vi "Begin.vi"(8 "error in":errorcluster) -> (0 "error out":errorcluster)   [LabVIEW 2018]
doc: "Called before other user functions, this VI is expected to open initial I/O refnums, load in file data, and do all program initialization. Notice that the <B>error out</B> terminal is simply used for data flow. Wiring it to other structures or subVIs ensures that this VI runs first."
uses:
  <vilib>/Rock Robotics/WPI/DriverStation/WPI_DriverStationRobotMode2.ctl
  <vilib>/Rock Robotics/WPI/Joystick/WPI_JoystickDeviceEnum.ctl
  <vilib>/Rock Robotics/WPI/Solenoid/WPI_SolenoidChannel.ctl
  <vilib>/Rock Robotics/WPI/ThirdParty/REV Robotics/SPARK MAX/Typedef/Spark MAX Motor Type.ctl
  <vilib>/Rock Robotics/WPI/ThirdParty/REV Robotics/SPARK MAX/Typedef/Spark MAX Limit Switch Polarity.ctl
  <vilib>/Rock Robotics/WPI/ThirdParty/REV Robotics/SPARK MAX/Typedef/Spark MAX Limit Direction.ctl
  <vilib>/Rock Robotics/WPI/ThirdParty/Phoenix-LabVIEW/Motor Controller/Controls/CTRE_Phoenix_MotorControl_FeedbackDevice.ctl
  <vilib>/Rock Robotics/WPI/ThirdParty/REV Robotics/SPARK MAX/Typedef/Spark MAX Idle Mode.ctl
  Robot Global Data.vi
  <vilib>/Rock Robotics/Network Tables/NT Write String Array.vi
  <vilib>/Rock Robotics/WPI/Solenoid/WPI_SolenoidOpenSingle.vi
  <vilib>/Rock Robotics/SystemInterfaces/DIO/FPGA_DIOPWMChannel.ctl
  <vilib>/Rock Robotics/WPI/SafetyOutput/WPI_SafetyOutputConfigMenu.ctl
  <vilib>/Rock Robotics/WPI/RobotDrive/WPI_RobotDriveOpen2MotorWithTalon.vi
panel:
  in  "FL F":dbl=0.000156
  in  "FL P":dbl=5e-05 format="%#_13g"
  in  "FR F":dbl=0.000156
  in  "FR P":dbl=5e-05 format="%#_13g"
  in  "BR F":dbl=0.000156
  in  "BR P":dbl=5e-05 format="%#_13g"
  in  "PID Constants Back Left Drive":T1={"P Gain"=2.5e-10, "I Gain"=0.0, "D Gain"=0.0, "F Gain"=0.000175, "I Zone"=0.0, "Min Output"=-1.0, "Max Output"=1.0}
  in  "PID Constants Front Right Drive":T1={"P Gain"=2.5e-10, "I Gain"=0.0, "D Gain"=0.0, "F Gain"=0.000175, "I Zone"=0.0, "Min Output"=-1.0, "Max Output"=1.0}
  in  "PID Constants Front Left Drive":T1={"P Gain"=2.5e-10, "I Gain"=0.0, "D Gain"=0.0, "F Gain"=0.000175, "I Zone"=0.0, "Min Output"=-1.0, "Max Output"=1.0}
  in  "PID Constants Back Right Drive":T1={"P Gain"=2.5e-10, "I Gain"=0.0, "D Gain"=0.0, "F Gain"=0.000175, "I Zone"=0.0, "Min Output"=-1.0, "Max Output"=1.0}
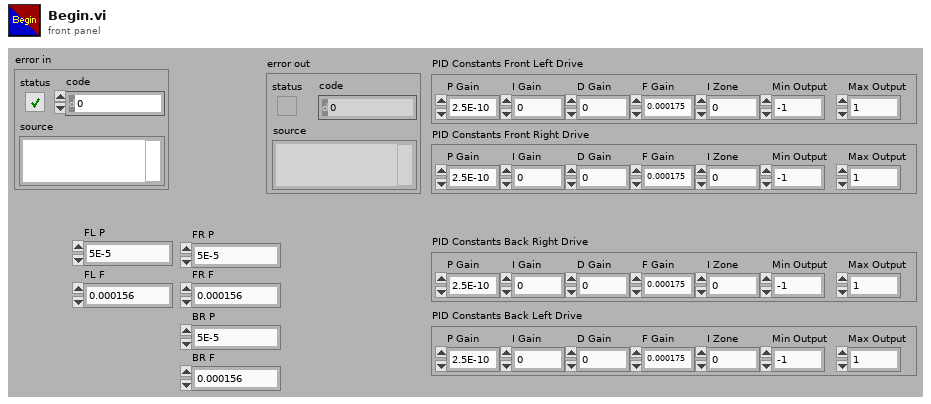
[diagram p1: front panel]
types:
  T1 = cluster{"P Gain":dbl, "I Gain":dbl, "D Gain":dbl, "F Gain":dbl, "I Zone":dbl, "Min Output":dbl, "Max Output":dbl}
  T2 = typedef "Spark MAX Idle Mode.ctl" = enum16{"Coast", "Brake"}
  T3 = typedef "Spark MAX Limit Direction.ctl" = enum16{"Forward Limit", "Reverse Limit"}
  T4 = typedef "Spark MAX Limit Switch Polarity.ctl" = enum16{"Normally Open", "Normally Closed"}
  T5 = typedef "CTRE_Phoenix_MotorControl_FeedbackDevice.ctl" = i8
  T6 = typedef "Spark MAX Motor Type.ctl" = enum16{"Brushed", "Brushless"}
  T7 = typedef "WPI_SolenoidChannel.ctl" = enum8{"Solenoid 0", "Solenoid 1", "Solenoid 2", "Solenoid 3", "Solenoid 4", "Solenoid 5", "Solenoid 6", "Solenoid 7", "Invalid"}
  T8 = typedef "WPI_JoystickDeviceEnum.ctl" = enum16{"USB 0", "USB 1", "USB 2", "USB 3", "USB 4", "USB 5"}
  T9 = typedef "WPI_DriverStationRobotMode2.ctl" = enum16{"Autonomous Disabled", "Autonomous Enabled", "Teleop Disabled", "Teleop Enabled", "Disconnected", "Finish", "Test Disabled", "Test Enabled", "Emergency Stopped"}
  T10 = typedef "WPI_SafetyOutputConfigMenu.ctl" = enum16{"Enable", "Disable"}
  T11 = typedef "FPGA_DIOPWMChannel.ctl" = enum8{"PWM 0", "PWM 1", "PWM 2", "PWM 3", "PWM 4", "PWM 5", "PWM 6", "PWM 7", "PWM 8", "PWM 9", "PWM MXP 0", "PWM MXP 1", "PWM MXP 2", "PWM MXP 3", "PWM MXP 4", "PWM MXP 5", "PWM MXP 6", "PWM MXP 7", "PWM MXP 8", "PWM MXP 9", "Invalid"}
  T12 = typedef "WPI_RobotDriveDevRef.ctl" = cluster{"DevStatus":errorcluster, "Motors[]":T13[], "Square Inputs":bool, "Max Output":dbl}
  T13 = typedef "WPI_MotorControlDeviceRef.ctl" = cluster{"DeviceStatus":errorcluster, "Type":T14, "PWM":cluster{"PWM Channel":T11, "DeadBand":T15}, "CAN":cluster{"Device Number":u8, "SetOutput VI Ref":variant, "GetOutput VI Ref":variant, "Enable VI Ref":variant, "Disable VI Ref":variant, "Data":variant}, "Invert":bool, "DIO PWM":cluster{"PWM \"Enable\" Channel":T11, "DIOChannel":T16, "PWM Rate":dbl}}
  T14 = typedef "WPI_MotorControlType.ctl" = enum16{"PWM", "CAN", "DIO PWM"}
  T15 = typedef "WPI_PWMDeadband.ctl" = cluster{"Name":string, "maxPositivePwm":i32, "minPositivePwm":i32, "centerPwm":i32, "maxNegativePwm":i32, "minNegativePwm":i32, "angularRange":u16}
  T16 = typedef "FPGA_DIOChannel.ctl" = enum8{"DIO 0", "DIO 1", "DIO 2", "DIO 3", "DIO 4", "DIO 5", "DIO 6", "DIO 7", "DIO 8", "DIO 9", "DIO MXP 0", "DIO MXP 1", "DIO MXP 2", "DIO MXP 3", "DIO MXP 4", "DIO MXP 5", "DIO MXP 6", "DIO MXP 7", "DIO MXP 8", "DIO MXP 9", "DIO MXP 10", "DIO MXP 11", "DIO MXP 12", "DIO MXP 13", "DIO MXP 14", "DIO MXP 15", "SPI Port CS1", "SPI Port CS2", "SPI Port CS3", "SPI Port MISO", "SPI Port MOSI", "Invalid"}
  T17 = typedef "WPI_JoystickDevRef.ctl" = cluster{"Device":T8}
  T18 = typedef "WPI_SolenoidDevRef.ctl" = cluster{"DevStatus":errorcluster, "Pneumatics Control Module":u8, "Forward Solenoid Channel":T7, "Reverse Solenoid Channel":T7}
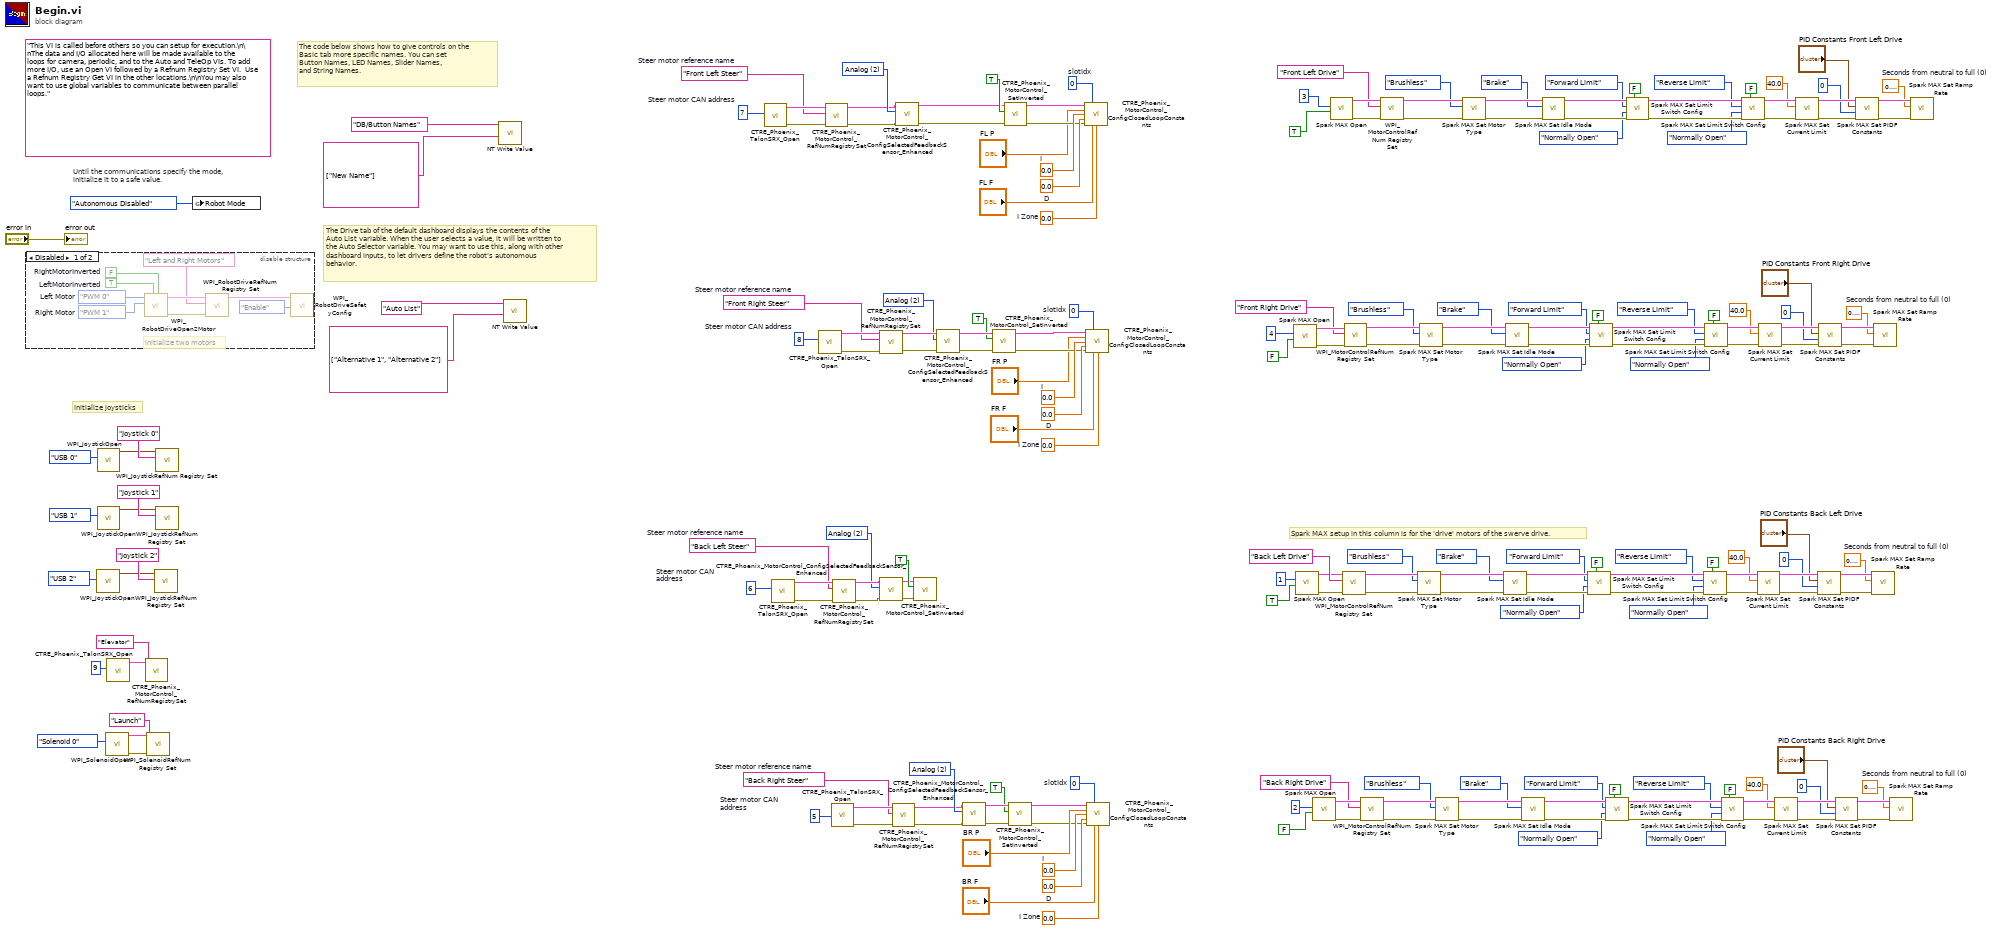
[diagram p0: block diagram]
diagram:
  w16 = sgl 0.2  # Seconds from neutral to full (0)
  w32 = T5 2 items=["QuadEncoder"=0, "Analog"=2, "Tachometer"=4, "Pulse Width Encoded Position"=8, "Sensor Sum (S0 + S1)"=9, "Sensor Difference (D0 - D1)"=10, "Remote Source 0"=11, "Remote Source 1"=12, "Software Emulated"=15] ("Feedback Device")
  w42 = 0.0  # I Zone
  w43 = 0.0  # D
  w44 = 0.0  # I
  w45 = 0  # slotIdx
  w40 = u8 8  # Steer motor CAN address
  w41 = "Front Right Steer"  # Steer motor reference name
  w57 = u8 5  # Steer motor CAN address
  w61 = T5 2 items=["QuadEncoder"=0, "Analog"=2, "Tachometer"=4, "Pulse Width Encoded Position"=8, "Sensor Sum (S0 + S1)"=9, "Sensor Difference (D0 - D1)"=10, "Remote Source 0"=11, "Remote Source 1"=12, "Software Emulated"=15] ("Feedback Device")
  w62 = 0.0  # I Zone
  w63 = 0.0  # D
  w64 = 0.0  # I
  w66 = 0  # slotIdx
  w27 = T5 2 items=["QuadEncoder"=0, "Analog"=2, "Tachometer"=4, "Pulse Width Encoded Position"=8, "Sensor Sum (S0 + S1)"=9, "Sensor Difference (D0 - D1)"=10, "Remote Source 0"=11, "Remote Source 1"=12, "Software Emulated"=15] ("Feedback Device")
  w80 = T5 2 items=["QuadEncoder"=0, "Analog"=2, "Tachometer"=4, "Pulse Width Encoded Position"=8, "Sensor Sum (S0 + S1)"=9, "Sensor Difference (D0 - D1)"=10, "Remote Source 0"=11, "Remote Source 1"=12, "Software Emulated"=15] ("Feedback Device")
  w81 = 0.0  # I Zone
  w82 = 0.0  # D
  w83 = 0.0  # I
  w84 = 0  # slotIdx
  w102 = sgl 0.2  # Seconds from neutral to full (0)
  w133 = sgl 0.2  # Seconds from neutral to full (0)
  w164 = sgl 0.2  # Seconds from neutral to full (0)
  w58 = "Back Right Steer"  # Steer motor reference name
  w69 = u8 6  # Steer motor CAN address
  w70 = "Back Left Steer"  # Steer motor reference name
  w77 = u8 7  # Steer motor CAN address
  w75 = "Front Left Steer"  # Steer motor reference name
  (unwired) "This VI is called before others so you can setup for execution.\n\nThe data and I/O allocated here will be made available to the loops for camera, periodic, and to the Auto and TeleOp VIs. To add more I/O, use an Open VI followed by a Refnum Registry Set VI.  Use a Refnum Registry Get VI in the other locations.\n\nYou may also want to use global variables to communicate between parallel loops."
  # "Spark MAX setup in this column is for the 'drive' motors of the swerve drive."
  # "The Drive tab of the default dashboard displays the contents of the\nAuto List variable. When the user selects a value, it will be written to\nthe Auto Selector variable. You may want to use this, along with other\ndashboard inputs, to let drivers define the robot's autonomous\nbehavior."
  # "The code below shows how to give controls on the\nBasic tab more specific names. You can set\nButton Names, LED Names, Slider Names,\nand String Names."
  # "initialize joysticks"
  # "Until the communications specify the mode,\ninitialize it to a safe value."
  n1 = disable-structure shown="Disabled" {
    frame Disabled {
      w213 = FPGA_DIOPWMChannel."PWM 1"  # Right Motor
      w214 = FPGA_DIOPWMChannel."PWM 0"  # Left Motor
      w218 = TRUE  # LeftMotorInverted
      w219 = FALSE  # RightMotorInverted
      # "initialize two motors"
      n2 = call-poly <vilib>:"WPI_RobotDriveOpen2Motor.vi"("Right Motor Inverted"=w219, "Left Motor Inverted"=w218, "Right Motor"=w213, "Left Motor"=w214) -> ("error out"=w215:errorcluster, "RobotDriveDevRef"=w217:T12)  [unwired: 1 in, 5 out]
      n3 = call <vilib>:"WPI_RobotDriveRefNum Registry Set.vi"("error in (no error)"=w215, "refnum name"="Left and Right Motors", "RobotDriveDevRef"=w217) -> ("RobotDriveDevRef"=w212:T12)  [unwired: 1 in, 7 out]
      n4 = call <vilib>:"WPI_RobotDriveSafetyConfig.vi"("mode"=WPI_SafetyOutputConfigMenu."Enable", "RobotDriveDevRef"=w212) -> ()  [unwired: 8 in, 2 out]
    }
    frame Enabled {
    }
  }
  n5 = call <vilib>:"WPI_JoystickOpen.vi"("JoystickDevice"=WPI_JoystickDeviceEnum."USB 2") -> ("JoystickDevRef"=w197:T17)  [unwired: 10 in]
  n6 = call <vilib>:"WPI_JoystickOpen.vi"("JoystickDevice"=WPI_JoystickDeviceEnum."USB 0") -> ("JoystickDevRef"=w208:T17)  [unwired: 10 in]
  n7 = call <vilib>:"WPI_JoystickOpen.vi"("JoystickDevice"=WPI_JoystickDeviceEnum."USB 1") -> ("JoystickDevRef"=w200:T17)  [unwired: 10 in]
  n8 = call-poly <vilib>:"WPI_SolenoidOpen.vi"("Solenoid Channel"=WPI_SolenoidChannel."Solenoid 0") -> ("error out"=w192:errorcluster, "SolenoidDevRef"=w191:T18)  [unwired: 9 in]
  n9 = call <vilib>:"CTRE_Phoenix_TalonSRX_Open.vi"("Device Number"=u8 9) -> ("CAN Talon SRX Ref"=w195:T13)  [unwired: 9 in, 1 out]
  n10 = call <vilib>:"CTRE_Phoenix_MotorControl_RefNumRegistrySet.vi"("refnum name"="Elevator", "PhoenixMotorControlDevRef"=w195) -> ()  [unwired: 8 in, 2 out]
  n11 = call <vilib>:"WPI_SolenoidRefNum Registry Set.vi"("error in (no error)"=w192, "refnum name"="Launch", "SolenoidDevRef"=w191) -> ()  [unwired: 7 in, 2 out]
  n12 = call <vilib>:"WPI_JoystickRefNum Registry Set.vi"("refnum name"="Joystick 2", "JoystickDevRef"=w197) -> ()  [unwired: 8 in, 2 out]
  n13 = call <vilib>:"WPI_JoystickRefNum Registry Set.vi"("refnum name"="Joystick 0", "JoystickDevRef"=w208) -> ()  [unwired: 8 in, 2 out]
  n14 = call <vilib>:"WPI_JoystickRefNum Registry Set.vi"("refnum name"="Joystick 1", "JoystickDevRef"=w200) -> ()  [unwired: 8 in, 2 out]
  n15 = global write "Robot Global Data.vi" "Robot Mode"(WPI_DriverStationRobotMode2."Autonomous Disabled" ("Robot Mode")) -> ()
  n16 = call-poly <vilib>:"NT Write Value.vi"("String Array"=string[] ["New Name"], "Name"="DB/Button Names") -> ()  [unwired: 9 in, 1 out]
  n17 = call-poly <vilib>:"NT Write Value.vi"("String Array"=string[] ["Alternative 1", "Alternative 2"], "Name"="Auto List") -> ()  [unwired: 9 in, 1 out]
  n18 = call <vilib>:"CTRE_Phoenix_TalonSRX_Open.vi"("Device Number"=w77) -> ("error out"=w85:errorcluster, "CAN Talon SRX Ref"=w76:T13)  [unwired: 9 in]
  n19 = call <vilib>:"CTRE_Phoenix_TalonSRX_Open.vi"("Device Number"=w69) -> ("error out"=w73:errorcluster, "CAN Talon SRX Ref"=w74:T13)  [unwired: 9 in]
  n20 = call <vilib>:"CTRE_Phoenix_TalonSRX_Open.vi"("Device Number"=w40) -> ("error out"=w46:errorcluster, "CAN Talon SRX Ref"=w47:T13)  [unwired: 9 in]
  n21 = call <vilib>:"CTRE_Phoenix_MotorControl_RefNumRegistrySet.vi"("error in (no error)"=w85, "refnum name"=w75, "PhoenixMotorControlDevRef"=w76) -> ("error out"=w78:errorcluster, "PhoenixMotorControlDevRef"=w79:T13)  [unwired: 7 in]
  n22 = call <vilib>:"CTRE_Phoenix_TalonSRX_Open.vi"("Device Number"=w57) -> ("error out"=w67:errorcluster, "CAN Talon SRX Ref"=w68:T13)  [unwired: 9 in]
  n23 = call <vilib>:"CTRE_Phoenix_MotorControl_RefNumRegistrySet.vi"("error in (no error)"=w73, "refnum name"=w70, "PhoenixMotorControlDevRef"=w74) -> ("error out"=w71:errorcluster, "PhoenixMotorControlDevRef"=w72:T13)  [unwired: 7 in]
  n24 = call <vilib>:"CTRE_Phoenix_MotorControl_RefNumRegistrySet.vi"("error in (no error)"=w46, "refnum name"=w41, "PhoenixMotorControlDevRef"=w47) -> ("error out"=w36:errorcluster, "PhoenixMotorControlDevRef"=w33:T13)  [unwired: 7 in]
  n25 = call <vilib>:"CTRE_Phoenix_MotorControl_ConfigSelectedFeedbackSensor_Enhanced.vi"("error in (no error)"=w71, "Feedback Device"=w27, "PhoenixMotorControlDevRef"=w72) -> ("error out"=w28:errorcluster, "PhoenixMotorControlDevRef"=w29:T13)  [unwired: 7 in]
  n26 = call <vilib>:"CTRE_Phoenix_MotorControl_RefNumRegistrySet.vi"("error in (no error)"=w67, "refnum name"=w58, "PhoenixMotorControlDevRef"=w68) -> ("error out"=w59:errorcluster, "PhoenixMotorControlDevRef"=w60:T13)  [unwired: 7 in]
  n27 = call <vilib>:"CTRE_Phoenix_MotorControl_ConfigSelectedFeedbackSensor_Enhanced.vi"("error in (no error)"=w78, "Feedback Device"=w80, "PhoenixMotorControlDevRef"=w79) -> ("error out"=w30:errorcluster, "PhoenixMotorControlDevRef"=w31:T13)  [unwired: 7 in]
  n28 = call <vilib>:"CTRE_Phoenix_MotorControl_SetInverted.vi"("error in (no error)"=w28, "Invert?"=TRUE, "PhoenixMotorControlDevRef"=w29) -> ()  [unwired: 7 in, 2 out]
  n29 = call <vilib>:"CTRE_Phoenix_MotorControl_ConfigSelectedFeedbackSensor_Enhanced.vi"("error in (no error)"=w36, "Feedback Device"=w32, "PhoenixMotorControlDevRef"=w33) -> ("error out"=w38:errorcluster, "PhoenixMotorControlDevRef"=w39:T13)  [unwired: 7 in]
  n30 = call <vilib>:"CTRE_Phoenix_MotorControl_ConfigSelectedFeedbackSensor_Enhanced.vi"("error in (no error)"=w59, "Feedback Device"=w61, "PhoenixMotorControlDevRef"=w60) -> ("error out"=w54:errorcluster, "PhoenixMotorControlDevRef"=w53:T13)  [unwired: 7 in]
  n31 = call <vilib>:"CTRE_Phoenix_MotorControl_SetInverted.vi"("error in (no error)"=w38, "Invert?"=TRUE, "PhoenixMotorControlDevRef"=w39) -> ("error out"=w35:errorcluster, "PhoenixMotorControlDevRef"=w34:T13)  [unwired: 7 in]
  n32 = call <vilib>:"CTRE_Phoenix_MotorControl_SetInverted.vi"("error in (no error)"=w30, "Invert?"=TRUE, "PhoenixMotorControlDevRef"=w31) -> ("error out"=w49:errorcluster, "PhoenixMotorControlDevRef"=w50:T13)  [unwired: 7 in]
  n33 = call <vilib>:"CTRE_Phoenix_MotorControl_SetInverted.vi"("error in (no error)"=w54, "Invert?"=TRUE, "PhoenixMotorControlDevRef"=w53) -> ("error out"=w55:errorcluster, "PhoenixMotorControlDevRef"=w56:T13)  [unwired: 7 in]
  n34 = call <vilib>:"CTRE_Phoenix_MotorControl_ConfigClosedLoopConstants.vi"("PhoenixMotorControlDevRef"=w50, "slotIdx"=w84, "P"="FL P", "I"=w83, "D"=w82, "error in (no error)"=w49, "F"="FL F", "I Zone"=w81) -> ()  [unwired: 6 in, 2 out]
  n35 = call <vilib>:"CTRE_Phoenix_MotorControl_ConfigClosedLoopConstants.vi"("PhoenixMotorControlDevRef"=w34, "slotIdx"=w45, "P"="FR P", "I"=w44, "D"=w43, "error in (no error)"=w35, "F"="FR F", "I Zone"=w42) -> ()  [unwired: 6 in, 2 out]
  n36 = call <vilib>:"CTRE_Phoenix_MotorControl_ConfigClosedLoopConstants.vi"("PhoenixMotorControlDevRef"=w56, "slotIdx"=w66, "P"="BR P", "I"=w64, "D"=w63, "error in (no error)"=w55, "F"="BR F", "I Zone"=w62) -> ()  [unwired: 6 in, 2 out]
  n37 = call <vilib>:"Spark MAX Open.vi"("Invert"=FALSE, "Device Number"=u8 4) -> ("error out"=w120:errorcluster, "MotorControlDeviceRef"=w121:T13)  [unwired: 8 in]
  n38 = call <vilib>:"Spark MAX Open.vi"("Invert"=TRUE, "Device Number"=u8 1) -> ("error out"=w87:errorcluster, "MotorControlDeviceRef"=w88:T13)  [unwired: 8 in]
  n39 = call <vilib>:"Spark MAX Open.vi"("Invert"=FALSE, "Device Number"=u8 2) -> ("error out"=w180:errorcluster, "MotorControlDeviceRef"=w182:T13)  [unwired: 8 in]
  n40 = call <vilib>:"Spark MAX Open.vi"("Invert"=TRUE, "Device Number"=u8 3) -> ("error out"=w151:errorcluster, "MotorControlDeviceRef"=w152:T13)  [unwired: 8 in]
  n41 = call <vilib>:"WPI_MotorControlRefNum Registry Set.vi"("error in (no error)"=w87, "refnum name"="Back Left Drive", "MotorControlDevRef"=w88) -> ("error out"=w113:errorcluster, "MotorControlDevRef"=w114:T13)  [unwired: 7 in]
  n42 = call <vilib>:"WPI_MotorControlRefNum Registry Set.vi"("error in (no error)"=w120, "refnum name"="Front Right Drive", "MotorControlDevRef"=w121) -> ("error out"=w144:errorcluster, "MotorControlDevRef"=w145:T13)  [unwired: 7 in]
  n43 = call <vilib>:"WPI_MotorControlRefNum Registry Set.vi"("error in (no error)"=w180, "refnum name"="Back Right Drive", "MotorControlDevRef"=w182) -> ("error out"=w187:errorcluster, "MotorControlDevRef"=w188:T13)  [unwired: 7 in]
  n44 = call <vilib>:"WPI_MotorControlRefNum Registry Set.vi"("error in (no error)"=w151, "refnum name"="Front Left Drive", "MotorControlDevRef"=w152) -> ("error out"=w175:errorcluster, "MotorControlDevRef"=w176:T13)  [unwired: 7 in]
  n45 = call <vilib>:"Spark MAX Set Motor Type.vi"("error in (no error)"=w113, "Enum"=Spark_MAX_Motor_Type."Brushless", "MotorControlDevRef"=w114) -> ("error out"=w111:errorcluster, "MotorControlDeviceRef"=w112:T13)  [unwired: 7 in]
  n46 = call <vilib>:"Spark MAX Set Motor Type.vi"("error in (no error)"=w144, "Enum"=Spark_MAX_Motor_Type."Brushless", "MotorControlDevRef"=w145) -> ("error out"=w142:errorcluster, "MotorControlDeviceRef"=w143:T13)  [unwired: 7 in]
  n47 = call <vilib>:"Spark MAX Set Motor Type.vi"("error in (no error)"=w187, "Enum"=Spark_MAX_Motor_Type."Brushless", "MotorControlDevRef"=w188) -> ("error out"=w185:errorcluster, "MotorControlDeviceRef"=w186:T13)  [unwired: 7 in]
  n48 = call <vilib>:"Spark MAX Set Motor Type.vi"("error in (no error)"=w175, "Enum"=Spark_MAX_Motor_Type."Brushless", "MotorControlDevRef"=w176) -> ("error out"=w173:errorcluster, "MotorControlDeviceRef"=w174:T13)  [unwired: 7 in]
  n49 = call <vilib>:"Spark MAX Set Idle Mode.vi"("error in (no error)"=w111, "Idle Mode"=Spark_MAX_Idle_Mode."Brake", "MotorControlDeviceRef in"=w112) -> ("error out"=w109:errorcluster, "MotorControlDeviceRef out"=w110:T13)  [unwired: 7 in]
  n50 = call <vilib>:"Spark MAX Set Idle Mode.vi"("error in (no error)"=w142, "Idle Mode"=Spark_MAX_Idle_Mode."Brake", "MotorControlDeviceRef in"=w143) -> ("error out"=w140:errorcluster, "MotorControlDeviceRef out"=w141:T13)  [unwired: 7 in]
  n51 = call <vilib>:"Spark MAX Set Idle Mode.vi"("error in (no error)"=w185, "Idle Mode"=Spark_MAX_Idle_Mode."Brake", "MotorControlDeviceRef in"=w186) -> ("error out"=w23:errorcluster, "MotorControlDeviceRef out"=w24:T13)  [unwired: 7 in]
  n52 = call <vilib>:"Spark MAX Set Idle Mode.vi"("error in (no error)"=w173, "Idle Mode"=Spark_MAX_Idle_Mode."Brake", "MotorControlDeviceRef in"=w174) -> ("error out"=w171:errorcluster, "MotorControlDeviceRef out"=w172:T13)  [unwired: 7 in]
  n53 = call <vilib>:"Spark MAX Set Limit Switch Config.vi"("Enabled? (T)"=FALSE, "error in (no error)"=w109, "Polarity (Normally Open)"=Spark_MAX_Limit_Switch_Polarity."Normally Open", "Limit Switch"=Spark_MAX_Limit_Direction."Forward Limit", "MotorControlDeviceRef in"=w110) -> ("error out"=w107:errorcluster, "MotorControlDeviceRef out"=w108:T13)  [unwired: 5 in]
  n54 = call <vilib>:"Spark MAX Set Limit Switch Config.vi"("Enabled? (T)"=FALSE, "error in (no error)"=w140, "Polarity (Normally Open)"=Spark_MAX_Limit_Switch_Polarity."Normally Open", "Limit Switch"=Spark_MAX_Limit_Direction."Forward Limit", "MotorControlDeviceRef in"=w141) -> ("error out"=w138:errorcluster, "MotorControlDeviceRef out"=w139:T13)  [unwired: 5 in]
  n55 = call <vilib>:"Spark MAX Set Limit Switch Config.vi"("Enabled? (T)"=FALSE, "error in (no error)"=w23, "Polarity (Normally Open)"=Spark_MAX_Limit_Switch_Polarity."Normally Open", "Limit Switch"=Spark_MAX_Limit_Direction."Forward Limit", "MotorControlDeviceRef in"=w24) -> ("error out"=w21:errorcluster, "MotorControlDeviceRef out"=w22:T13)  [unwired: 5 in]
  n56 = call <vilib>:"Spark MAX Set Limit Switch Config.vi"("Enabled? (T)"=FALSE, "error in (no error)"=w171, "Polarity (Normally Open)"=Spark_MAX_Limit_Switch_Polarity."Normally Open", "Limit Switch"=Spark_MAX_Limit_Direction."Forward Limit", "MotorControlDeviceRef in"=w172) -> ("error out"=w169:errorcluster, "MotorControlDeviceRef out"=w170:T13)  [unwired: 5 in]
  n57 = call <vilib>:"Spark MAX Set Limit Switch Config.vi"("Enabled? (T)"=FALSE, "error in (no error)"=w107, "Polarity (Normally Open)"=Spark_MAX_Limit_Switch_Polarity."Normally Open", "Limit Switch"=Spark_MAX_Limit_Direction."Reverse Limit", "MotorControlDeviceRef in"=w108) -> ("error out"=w116:errorcluster, "MotorControlDeviceRef out"=w115:T13)  [unwired: 5 in]
  n58 = call <vilib>:"Spark MAX Set Limit Switch Config.vi"("Enabled? (T)"=FALSE, "error in (no error)"=w138, "Polarity (Normally Open)"=Spark_MAX_Limit_Switch_Polarity."Normally Open", "Limit Switch"=Spark_MAX_Limit_Direction."Reverse Limit", "MotorControlDeviceRef in"=w139) -> ("error out"=w147:errorcluster, "MotorControlDeviceRef out"=w146:T13)  [unwired: 5 in]
  n59 = call <vilib>:"Spark MAX Set Limit Switch Config.vi"("Enabled? (T)"=FALSE, "error in (no error)"=w21, "Polarity (Normally Open)"=Spark_MAX_Limit_Switch_Polarity."Normally Open", "Limit Switch"=Spark_MAX_Limit_Direction."Reverse Limit", "MotorControlDeviceRef in"=w22) -> ("error out"=w26:errorcluster, "MotorControlDeviceRef out"=w25:T13)  [unwired: 5 in]
  n60 = call <vilib>:"Spark MAX Set Limit Switch Config.vi"("Enabled? (T)"=FALSE, "error in (no error)"=w169, "Polarity (Normally Open)"=Spark_MAX_Limit_Switch_Polarity."Normally Open", "Limit Switch"=Spark_MAX_Limit_Direction."Reverse Limit", "MotorControlDeviceRef in"=w170) -> ("error out"=w178:errorcluster, "MotorControlDeviceRef out"=w177:T13)  [unwired: 5 in]
  n61 = call <vilib>:"Spark MAX Set Current Limit.vi"("error in (no error)"=w116, "Current Limit A (100)"=sgl 40.0, "MotorControlDeviceRef in"=w115) -> ("error out"=w105:errorcluster, "MotorControlDeviceRef out"=w106:T13)  [unwired: 7 in]
  n62 = call <vilib>:"Spark MAX Set Current Limit.vi"("error in (no error)"=w147, "Current Limit A (100)"=sgl 40.0, "MotorControlDeviceRef in"=w146) -> ("error out"=w136:errorcluster, "MotorControlDeviceRef out"=w137:T13)  [unwired: 7 in]
  n63 = call <vilib>:"Spark MAX Set Current Limit.vi"("error in (no error)"=w26, "Current Limit A (100)"=sgl 40.0, "MotorControlDeviceRef in"=w25) -> ("error out"=w19:errorcluster, "MotorControlDeviceRef out"=w20:T13)  [unwired: 7 in]
  n64 = call <vilib>:"Spark MAX Set Current Limit.vi"("error in (no error)"=w178, "Current Limit A (100)"=sgl 40.0, "MotorControlDeviceRef in"=w177) -> ("error out"=w167:errorcluster, "MotorControlDeviceRef out"=w168:T13)  [unwired: 7 in]
  n65 = call <vilib>:"Spark MAX Set PIDF Constants.vi"("error in"=w105, "PIDF Slot"=0, "PID Constants"="PID Constants Back Left Drive", "MotorControlDeviceRef"=w106) -> ("error out"=w103:errorcluster, "MotorControlDeviceRef"=w104:T13)  [unwired: 6 in]
  n66 = call <vilib>:"Spark MAX Set PIDF Constants.vi"("error in"=w136, "PIDF Slot"=0, "PID Constants"="PID Constants Front Right Drive", "MotorControlDeviceRef"=w137) -> ("error out"=w134:errorcluster, "MotorControlDeviceRef"=w135:T13)  [unwired: 6 in]
  n67 = call <vilib>:"Spark MAX Set PIDF Constants.vi"("error in"=w19, "PIDF Slot"=0, "PID Constants"="PID Constants Back Right Drive", "MotorControlDeviceRef"=w20) -> ("error out"=w17:errorcluster, "MotorControlDeviceRef"=w18:T13)  [unwired: 6 in]
  n68 = call <vilib>:"Spark MAX Set PIDF Constants.vi"("error in"=w167, "PIDF Slot"=0, "PID Constants"="PID Constants Front Left Drive", "MotorControlDeviceRef"=w168) -> ("error out"=w165:errorcluster, "MotorControlDeviceRef"=w166:T13)  [unwired: 6 in]
  n69 = call <vilib>:"Spark MAX Set Ramp Rate.vi"("error in (no error)"=w103, "Seconds from neutral to full (0)"=w102, "MotorControlDeviceRef in"=w104) -> ()  [unwired: 7 in, 2 out]
  n70 = call <vilib>:"Spark MAX Set Ramp Rate.vi"("error in (no error)"=w134, "Seconds from neutral to full (0)"=w133, "MotorControlDeviceRef in"=w135) -> ()  [unwired: 7 in, 2 out]
  n71 = call <vilib>:"Spark MAX Set Ramp Rate.vi"("error in (no error)"=w17, "Seconds from neutral to full (0)"=w16, "MotorControlDeviceRef in"=w18) -> ()  [unwired: 7 in, 2 out]
  n72 = call <vilib>:"Spark MAX Set Ramp Rate.vi"("error in (no error)"=w165, "Seconds from neutral to full (0)"=w164, "MotorControlDeviceRef in"=w166) -> ()  [unwired: 7 in, 2 out]
  "error out" <- "error in"
